vi "64IN_1 WaitInId.vi"(6 "time(0.1)":i32=100, 8 "error in":errorcluster, 9 "Wait?":bool=TRUE, 10 "Status":bool, 11 "64IIN_1 Select":T1) -> (0 "error Out":errorcluster, 2 "TimeOut":bool, 3 "StatusOut":bool)   [LabVIEW 2019]
uses:
  Ctrl/64In_1 SelectInPut.ctl
  global/InAndOutGB.vi
  global/IO_FlagGB.vi
panel:
  # "64IN_1"
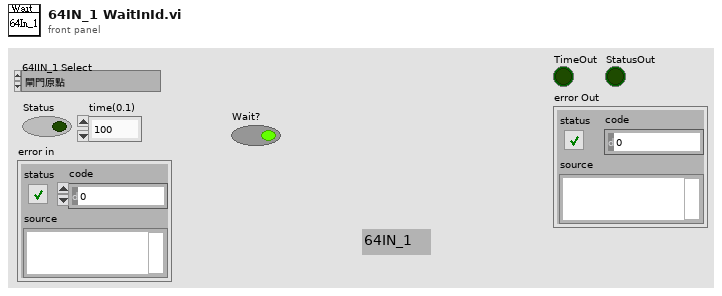
[diagram p1: front panel]
types:
  T1 = typedef "64In_1 SelectInPut.ctl" = enum16{"閘門原點", "閘門進點", "翻轉原點", "翻轉進點", "左入料檢知", "右入料檢知", "翻轉滿料檢知", "UBE#1", "UBE#2", "探針原點_1", "探針進點_1", "UBE#14", "UBE#13", "Scanner讀取OK", "Scanner讀取NG", "Scanner Busy", "儀器完成", "電池旋轉移載原點", "電池旋轉移載進點", "UBE#5", "UBE#6", "不良品分料原點", "不良品分料進點", "不良品分層原點", "不良品分層進點", "上層載台有無感知", "上層不良品滿料感知", "下層不良品箱到位感知", "上層不良品軌道滿料感知", "下層不良品滿料感知", "UBE#7", "UBE#8", "不良品排出氣缸原點", "不良品排出氣缸進點", "轉輪滿料檢知", "轉輪進料檢知", "良品出料檢知", "未出料檢知", "UBE#9", "UBE#10", "推出氣缸原點_1", "推出氣缸進點_1", "推出氣缸原點_2", "推出氣缸進點_2", "推出氣缸原點_3", "推出氣缸進點_3", "推出氣缸原點_4", "推出氣缸進點_4", "推出氣缸原點_5", "推出氣缸進點_5", "推出氣缸原點_6", "推出氣缸進點_6", "推出氣缸原點_7", "推出氣缸進點_7", "移載到位感知", "末端產品有無感知", "UBE#11", "氣壓檢知", "緊急停止", "收料復歸按鈕", "進料升降汽缸原點", "進料升降汽缸進點", "放料汽缸進點", "放料汽缸原點"}
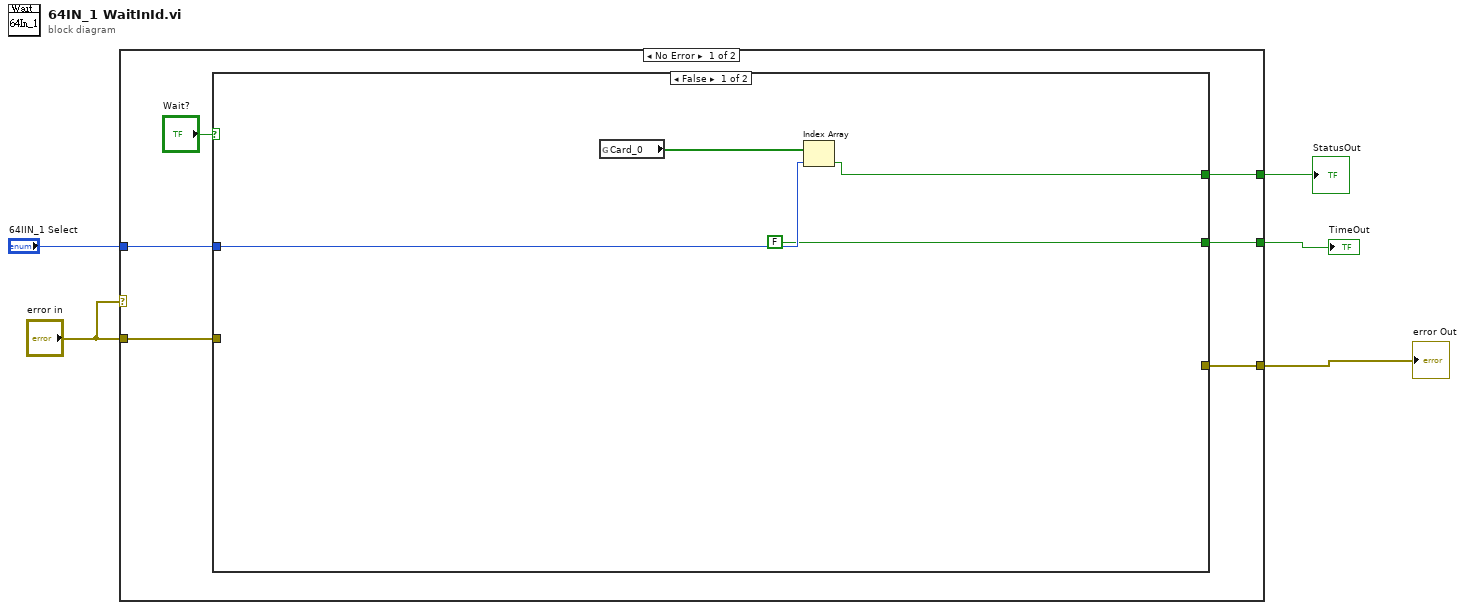
[diagram p0: block diagram]
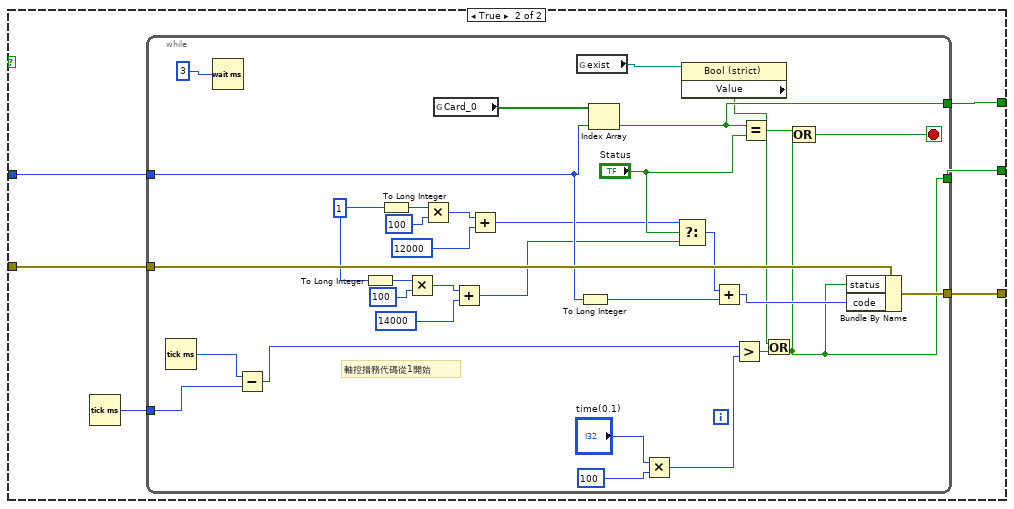
[diagram p2: hidden frame]
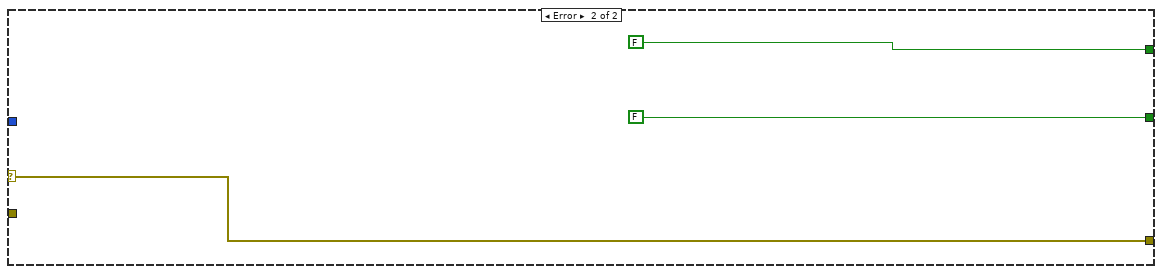
[diagram p3: hidden frame]
diagram:
  n1 = case shown="No Error" "error in" {
    selector: "error in" -> [_ w56]
    tunnel: [w11 FALSE] -> w5
    tunnel: "error in" -> [w10 _]
    tunnel: [w9 w56] -> w4
    tunnel: [w8 FALSE ("Boolean")] -> w2
    tunnel: "64IIN_1 Select" -> [w6 _]
    frame No Error {
      n2 = case shown="False" "Wait?" {
        tunnel: [FALSE w21] -> w11
        tunnel: w10 -> [_ w20]
        tunnel: [_ w19] -> w9
        tunnel: [w14 w18] -> w8
        tunnel: w6 -> [w15 w17]
        frame False {
          n3 = global read "InAndOutGB.vi" "Card_0"() -> (w12:bool[])
          n4 = Index Array(array=w12, index=w15) -> (element=w14:bool)
        }
        frame True {
          n5 = Tick Count (ms)() -> (millisecond timer value=w16:u32)
          n6 = while {
            tunnel: [w43] -> w21
            tunnel: w20 -> [w50]
            tunnel: [w47] -> w19
            tunnel: [w42] -> w18
            tunnel: w17 -> [w40]
            tunnel: w16 -> [w24]
            stop <- w52 stop-if-true
            w22 = 1 ("number")
            # "軸控措務代碼從1開始"
            n7 = Tick Count (ms)() -> (millisecond timer value=w25:u32)
            n8 = Wait (ms)(milliseconds to wait=u32 3) -> ()  [unwired: 1 out]
            n9 = Subtract(x=w25, y=w24) -> (x-y=w23:u32)
            n10 = To Long Integer(number=w22) -> (32bit integer=w30:i32)
            n11 = To Long Integer(number=w22) -> (32bit integer=w38:i32)
            n12 = Multiply(x=w30, y=100) -> (x*y=w32:i32)
            n13 = Multiply(x=w38, y=100) -> (x*y=w36:i32)
            n14 = global read "InAndOutGB.vi" "Card_0"() -> (w53:bool[])
            n15 = Add(x=w32, y=14000) -> (x+y=w29:i32)
            n16 = Add(x=w36, y=12000) -> (x+y=w34:i32)
            n17 = global read "IO_FlagGB.vi" "exist"() -> (w39:refnum<vi>)
            n18 = To Long Integer(number=w40) -> (32bit integer=w44:i32)
            n19 = Index Array(array=w53, index=w40) -> (element=w42:bool)
            n20 = Multiply(x="time(0.1)", y=u32 100 ("milliseconds to wait")) -> (x*y=w26:u32)
            n21 = Select(t=w34, s="Status", f=w29) -> (s? t:f=w45:i32)
            n22 = property class="Bool (strict)"(reference=w39) -> ("Value"=w41:bool)  [unwired: 1 in, 2 out]
            n23 = Add(x=w45, y=w44) -> (x+y=w48:i32)
            n24 = Greater?(x=w23, y=w26) -> (0:w49:bool)
            n25 = Equal?(x=w42, y="Status") -> (x = y?=w51:bool)
            n26 = Or(x=w41, y=w49) -> (x .or. y?=w43:bool)
            n27 = Compound Arithmetic op=OR(w51, w43) -> (w52:bool)
            n28 = Bundle By Name(cluster=w50, "status"=w43, "code"=w48) -> (w47:errorcluster)
          }
        }
      }
    }
    frame Error {
    }
  }
  "TimeOut" <- w5
  "error Out" <- w4
  "StatusOut" <- w2
